vi "NI VeriStand - Get Custom Device Decimation.vi"(8 "error in (no error)":errorcluster, 11 "Device Ref in":T1 format="%.0x") -> (0 "error out":errorcluster, 2 "Decimation":i32, 3 "Device Ref out":T1 format="%.0x")   [LabVIEW 2020, in "Custom Device API.lvlib"]
doc: "Returns the <B>Decimation</B> of a custom device, which determines how many iterations of the Primary Control Loop occur between calls to the custom device. A value of 1 indicates no decimation."
uses:
  <vilib>/NI VeriStand/Custom Device API/Custom Device API.lvlib
  <vilib>/NI VeriStand/Custom Device API/Custom Device Item Ref.ctl
  2da0e768-3996-47bb-a2a8-7c37467c956d.vi
  <vilib>/NI VeriStand/Custom Device API/Custom Device Offline Path.vi
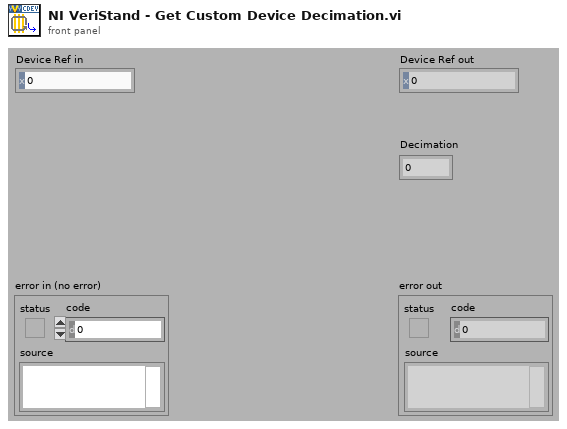
[diagram p1: front panel]
types:
  T1 = typedef "Custom Device API.lvlib/Custom Device Item Ref.ctl" = u64
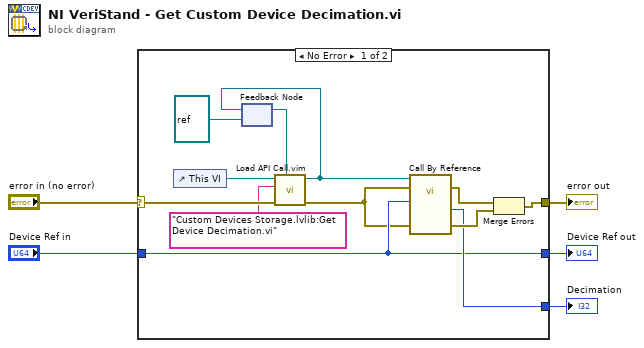
[diagram p0: block diagram]
diagram:
  n1 = case shown="No Error" "error in (no error)" {
    selector: "error in (no error)" -> [w11 w19]
    tunnel: "Device Ref in" -> [w14 w18]
    tunnel: [w16 w19] -> w4
    tunnel: [w14 w18] -> w3
    tunnel: [w15 _] -> w2
    frame No Error {
      n2 = control-ref of="This VI"() -> (w12:refnum<vi>)
      n3 = feedback #1(refnum<vi> refnum ("type specifier VI Refnum (for type only)")) -> (w13:refnum<vi>)
      n4 = call "Load API Call.vim"("VI reference in"=w13, "error in (no error)"=w11, "VI qualified name"="Custom Devices Storage.lvlib:Get Device Decimation.vi", "Caller VI ref"=w12) -> ("error out"=w9:errorcluster, "VI reference"=w10:refnum<vi>)  [unwired: 6 in]
      n5 = feedback-in #1(w10) -> ()
      n6 = call-by-ref "?"(reference=w10, error in=w9, 8:"error in (no error)"=w9, "Device Ref in"=w14) -> (error out=w6:errorcluster, 0:"error out"=w17:errorcluster, "Decimation"=w15:i32)  [unwired: 7 in, 2 out]
      n7 = Merge Errors(w6, w17) -> (w16:errorcluster)
    }
    frame Error {
    }
  }
  "Device Ref out" <- w3
  "error out" <- w4
  "Decimation" <- w2
